vi "close MB.vi"(8 "error in (no error)":errorcluster caption="错误输入（无错误）", 11 "HL7 输入":refnum<class "HL7.lvclass">) -> (0 "error out":errorcluster caption="错误输出", 3 "HL7 输出":refnum<class "HL7.lvclass">)   [LabVIEW 2016, in "HL7.lvlib" / "HL7.lvclass"]
uses:
  HL7.lvclass
  <vilib>/Plasmionique/MB Master/MB_Master/MB_Master.lvclass
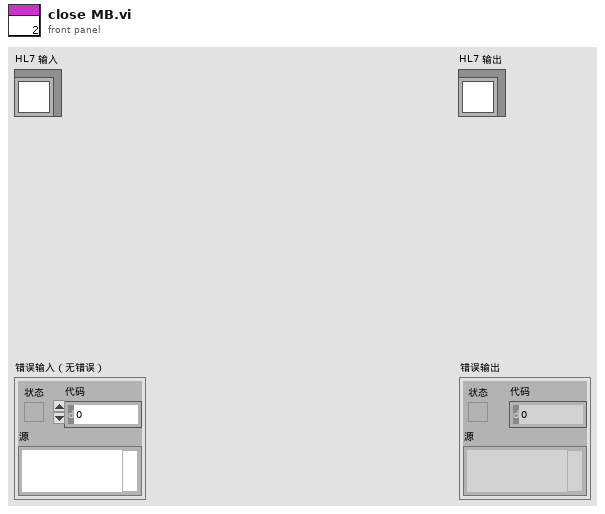
[diagram p1: front panel]
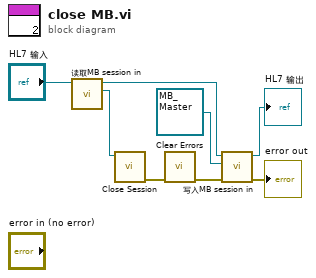
[diagram p0: block diagram]
diagram:
  n1 = call-dynamic "读取MB session in.vi"("HL7输入"="HL7 输入") -> ("MB Serial Master:MB_Master"=w7:refnum<class "MB_Master.lvclass">, "HL7输出"=w5:refnum<class "HL7.lvclass">)  [unwired: 8 in, 1 out]
  n2 = call-dynamic "Close Session.vi"("MB session in"=w7) -> ("error out"=w6:errorcluster)  [unwired: 10 in]
  n3 = call <vilib>:"Clear Errors.vi"("error in (no error)"=w6) -> ("error out"=w3:errorcluster)  [unwired: 5 in, 1 out]
  n4 = call-dynamic "写入MB session in.vi"("error in (no error)"=w3, "MB Serial Master:MB_Master"=refnum<class "MB_Master.lvclass"> refnum, "HL7输入"=w5) -> ("error out"=→"error out":errorcluster, "HL7输出"=→"HL7 输出":refnum<class "HL7.lvclass">)  [unwired: 7 in]
